vi "PTSequencer.swap steps.vi"(0 "i ref in":refnum<vi>, 2 "old indexes":i32[](array[numeric]), 3 "ms timeout (10000)":i32=10000, 4 "new indexes":i32[](array[numeric]), 5 "error in (no error)":errorcluster) -> (14 "i ref out":refnum<vi>, 17 "timed out":bool, 19 "error out":errorcluster)   [LabVIEW 2014, in "PTSequencer.lvlib"]
uses:
  PTSequencer.lvlib
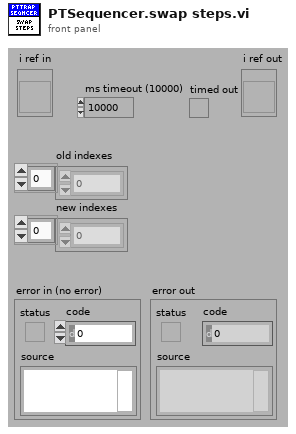
[diagram p1: front panel]
types:
  T1 = typedef "PTSequencer.lvlib/PTSequencer.i attribute.ctl" = cluster{"subsequence":bool, "mode":T2, "i step":i32, "nofLoops":i32, "i loop":i32, "Running":bool, "Paused":bool, "step done":bool, "loop done":bool, "seq done":bool, "DIM IDs":cluster{"step done":i32, "loop done":i32, "seq done":i32, "i step":i32, "i loop":i32}, "use stop conditions":bool, "stop conditions":T3[], "Step List":T5[], "DIM subsriptions":string[], "stop cond indexes":i32[], "step cond indexes":cluster{"step condition IDs":cluster{"step ID":i32, "condition ID":i32}[]}[], "Delay Start Time":timestamp, "status":string, "stopping":bool}
  T2 = typedef "PTSequencer.lvlib/PTSequencer.mode.ctl" = enum16{"single", "loop", "for loop"}
  T3 = typedef "PTSequencer.lvlib/PTSequencer.DIM service condition.ctl" = cluster{"DIM service":string, "descr":string, "nomValue":T4, "actValue":T4, "matched":bool, "DIM Status":cluster{"no link":bool, "quality":i32, "Time Stamp":timestamp}}
  T4 = typedef "CoreDefs.rawDataType.ctl" = i8[]
  T5 = typedef "PTSequencer.lvlib/PTSequencer.step.ctl" = cluster{"description":string, "object parameters":cluster{"object":string, "selector":string, "descriptor":string, "data":T4, "subsequence":bool, "call mode":enum16{"Simple DIM", "Synchronous"}, "data in":T4}, "result action":cluster{"check":bool, "passed":enum16{"Next", "Previous", "Repeat", "Jump"}, "failed":enum16{"Next", "Previous", "Repeat", "Jump"}, "jumpID_passed":i32, "jumpID_failed":i32}, "conditions":T3[], "fulfilled ":bool, "use delay":bool, "delay time (s)":dbl, "ID":i32}
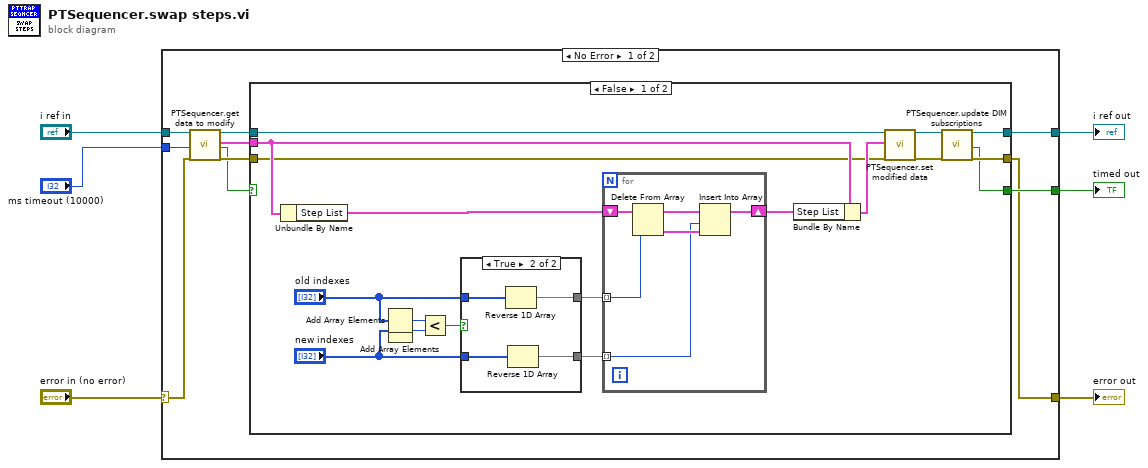
[diagram p0: block diagram]
diagram:
  n1 = case shown="No Error" "error in (no error)" {
    selector: "error in (no error)" -> [w13 w50]
    tunnel: "i ref in" -> [w16 w51]
    tunnel: [w7 w51] -> w5
    tunnel: "ms timeout (10000)" -> [w10 _]
    tunnel: [w9 _] -> w2
    tunnel: [w8 w50] -> w1
    frame No Error {
      n2 = call "PTSequencer.get data to modify.vi"("i ref in"=w16, "ms timeout (10000)"=w10, "error in (no error)"=w13) -> ("i ref out"=w15:refnum<vi>, "i attribute"=w14:T1, "timed out"=w11:bool, "error out"=w12:errorcluster)  [unwired: 13 in]
      n3 = case shown="False" w11 {
        selector: w11 -> [_ w47]
        tunnel: w15 -> [w34 w48]
        tunnel: [w19 w48] -> w7
        tunnel: w14 -> [w32 _]
        tunnel: w12 -> [w31 w49]
        tunnel: [w18 w49] -> w8
        tunnel: [w17 w47] -> w9
        frame False {
          n4 = Unbundle By Name(w32) -> ("Step List"=w25:T5[])
          n5 = Add Array Elements(numeric array="old indexes") -> (sum=w30:i32)
          n6 = Add Array Elements(numeric array="new indexes") -> (sum=w29:i32)
          n7 = Less?(x=w30, y=w29) -> (x < y?=w28:bool)
          n8 = case shown="True" w28 {
            tunnel: "new indexes" -> [w35 w40]
            tunnel: [w35 w39] -> w27
            tunnel: "old indexes" -> [w36 w38]
            tunnel: [w36 w37] -> w26
            frame False {
            }
            frame True {
              n9 = Reverse 1D Array(array=w38) -> (reversed array=w37:i32[])
              n10 = Reverse 1D Array(array=w40) -> (reversed array=w39:i32[])
            }
          }
          n11 = for {
            shift-right: [w43] -> w24
            shift-left: w25 -> [w46]
            tunnel: w27 -> [w41] mode=indexing
            tunnel: w26 -> [w42] mode=indexing
            n12 = Delete From Array(array=w46, index=w42) -> (deleted portion=w44:T5, array with subset deleted=w45:T5[])  [unwired: 1 in]
            n13 = Insert Into Array(array=w45, index=w41, new element=w44) -> (w43:T5[])
          }
          n14 = Bundle By Name(cluster=w32, "Step List"=w24) -> (w33:T1)
          n15 = call "PTSequencer.set modified data.vi"("i ref in"=w34, "CLASS.i attribute"=w33, "error in (no error)"=w31) -> ("i ref out"=w20:refnum<vi>, "error out"=w21:errorcluster)  [unwired: 15 in]
          n16 = call "PTSequencer.update DIM subscriptions.vi"("i ref in"=w20, "error in"=w21) -> ("i ref out"=w19:refnum<vi>, "timed out"=w17:bool, "error out"=w18:errorcluster)  [unwired: 15 in]
        }
        frame True {
        }
      }
    }
    frame Error {
    }
  }
  "error out" <- w1
  "i ref out" <- w5
  "timed out" <- w2
